vi "GetCellStrColor.vi"(7 "Color":u32, 8 "error in (no error)":errorcluster, 10 "Hdr Name":T1, 11 "Frequency in":refnum<class "Frequency.lvclass">) -> (0 "error out":errorcluster, 1 "Cell String":string, 2 "Cell Color":u32, 3 "Frequency out":refnum<class "Frequency.lvclass">)   [LabVIEW 2012, in "Measurement Channels.lvlib" / "Frequency.lvclass"]
uses:
  Frequency.lvclass
  Common/Controls/HeaderNames.ctl
  Class Voltage/Voltage.lvclass
  SubVIs Table/Custom Ctls Table/ge_ColType.ctl
  Frequency.lvclass/Frequency.ctl
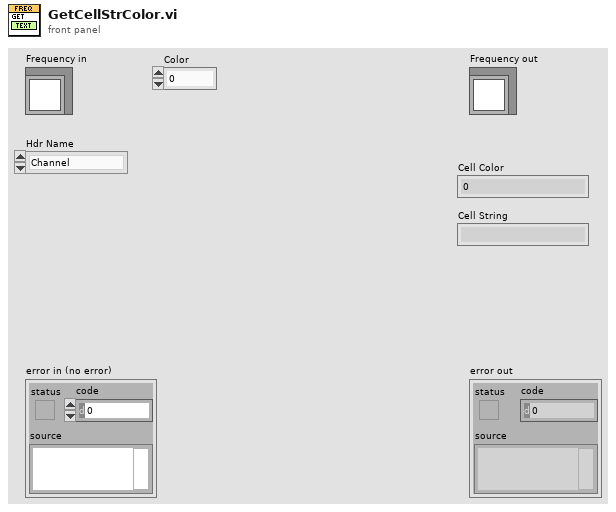
[diagram p1: front panel]
types:
  T1 = typedef "HeaderNames.ctl" = enum16{"Channel", "Device", "Spacer", "Description", "MB", "Range", "Terminal", "Coupling", "Thresh (V)", "Pulse/Rev", "Slope", "Min EU", "Min RPM", "mV/EU", "Iex", "Temp Units", "Type", "CJC Src", "CJC Val", "Ro", "Wire Cfg", "Strain Mode", "Vex", "Bridge Type", "GF", "Gauge Res", "Poisson", "Lead Res", "Init Strain", "GAF", "Scale", "Offset", "Unit (EU)", "dB?", "dB Ref", "Cal Mag", "Cal Units", "Max Temp", "Min Temp", "Max Strain", "Min Strain"}
  T2 = typedef "ge_ColType.ctl" = enum16{"Volts", "Amps", "Ohms", "TermCfg", "WireCfg", "Coup", "Slope", "Iex", "CalUnits", "ThrmUnits", "ThrmType", "CJCSrc", "BrdgType", "Strn Mode", "RTDType"}
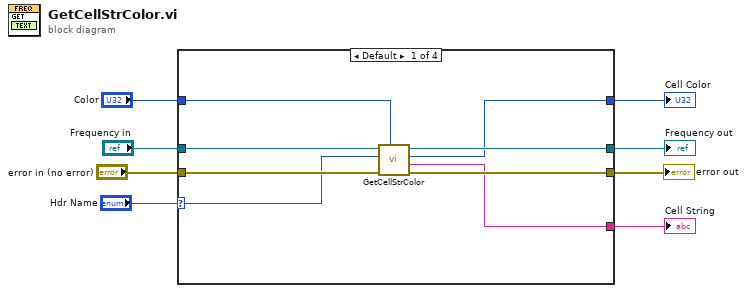
[diagram p0: block diagram]
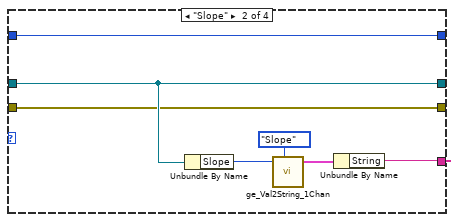
[diagram p2: hidden frame]
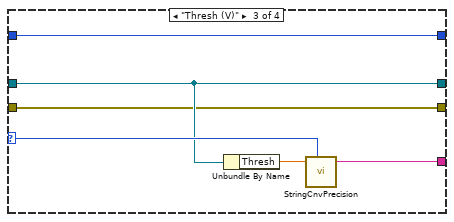
[diagram p3: hidden frame]
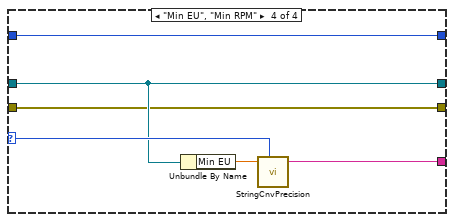
[diagram p4: hidden frame]
diagram:
  n1 = case shown="Default" "Hdr Name" {
    selector: "Hdr Name" -> [w9 _ w27 w33]
    tunnel: "Frequency in" -> [w16 w18 w26 w32]
    tunnel: [w12 w20 w28 w34] -> w6
    tunnel: [w11 w19 w24 w30] -> w5
    tunnel: "Color" -> [w10 w19 w24 w30]
    tunnel: [w14 w18 w26 w32] -> w7
    tunnel: "error in (no error)" -> [w15 w17 w25 w31]
    tunnel: [w13 w17 w25 w31] -> w1
    frame Default {
      n2 = call-parent "GetCellStrColor.vi"("Color"=w10, "error in (no error)"=w15, "Hdr Name"=w9, "Voltage in"=w16) -> ("error out"=w13:errorcluster, "Cell String"=w12:string, "Cell Color"=w11:u32, "Voltage out"=w14:refnum<class "Frequency.lvclass">)  [unwired: 4 in]
    }
    frame "Slope" {
      n3 = Unbundle By Name(w18) -> ("Slope"=w21:u16)
      n4 = call "ge_Val2String_1Chan.vi"("Value"=w21, "ColType"=ge_ColType."Slope") -> ("String and Val"=w22:cluster{"String":string, "Value":u16})  [unwired: 5 in]
      n5 = Unbundle By Name(w22) -> ("String"=w20:string)
    }
    frame "Thresh (V)" {
      n6 = Unbundle By Name(w26) -> ("Thresh"=w29:dbl)
      n7 = call "StringCnvPrecision.vi"("Number"=w29, "Header"=w27) -> ("Float String"=w28:string)  [unwired: 5 in]
    }
    frame "Min EU", "Min RPM" {
      n8 = Unbundle By Name(w32) -> ("Min EU"=w35:dbl)
      n9 = call "StringCnvPrecision.vi"("Number"=w35, "Header"=w33) -> ("Float String"=w34:string)  [unwired: 5 in]
    }
  }
  "error out" <- w1
  "Frequency out" <- w7
  "Cell String" <- w6
  "Cell Color" <- w5
